vi "Airmar open and config serial port.vi"(8 "error in (no error)":errorcluster, 9 "Input\nbuffer size":u32=4096, 10 "baud rate":u32=4800, 11 "VISA Refnum in":refnum<visa-resource-name>) -> (0 "error out":errorcluster, 3 "VISA Refnum out":refnum<visa-resource-name>)   [LabVIEW 2013]
doc: "opens a serial port (on the RIO or a standard computer) and sets up the buffers so they actually work.\n-Jason"
uses:
  <vilib>/Instr/_visa.llb/VISA Configure Serial Port (Instr).vi
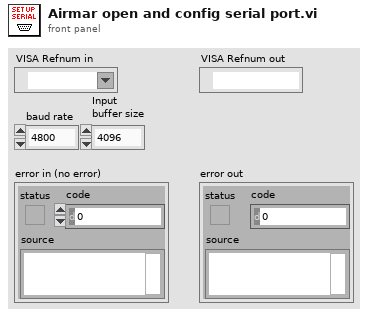
[diagram p1: front panel]
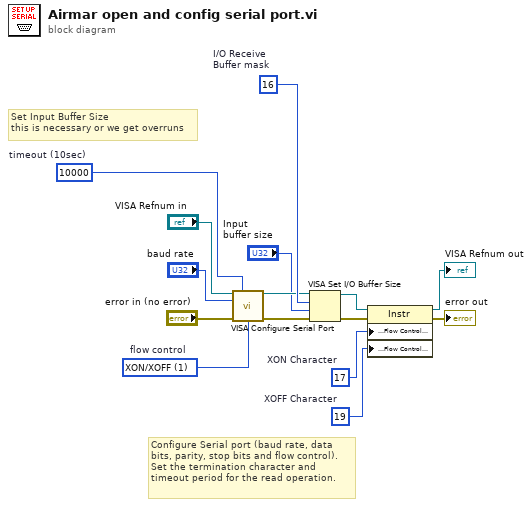
[diagram p0: block diagram]
diagram:
  w10 = u32 10000  # timeout (10sec)
  w7 = u8 19  # XOFF Character
  w6 = u8 17  # XON Character
  w11 = u16 16  # I/O Receive Buffer mask
  w2 = u16 1 items=["None"=0, "XON/XOFF"=1, "RTS/CTS"=2, "DTR/DSR"=4]  # flow control
  # "Set Input Buffer Size\nthis is necessary or we get overruns"
  # "Configure Serial port (baud rate, data\nbits, parity, stop bits and flow control).\nSet the termination character and\ntimeout period for the read operation."
  n1 = call-poly "VISA Configure Serial Port"("VISA resource name"="VISA Refnum in", "timeout (10sec)"=w10, "baud rate (9600)"="baud rate", "error in (no error)"="error in (no error)", "flow control (0:none)"=w2) -> ("VISA resource name out"=w8:refnum<visa-resource-name>, "error out"=w9:errorcluster)  [unwired: 9 in]
  n2 = VISA Set I/O Buffer Size(VISA resource name=w8, mask (16)=w11, size (4096)="Input\nbuffer size", error in (no error)=w9) -> (VISA resource name out=w4:refnum<visa-resource-name>, error out=w5:errorcluster)
  n3 = property class="Instr"(reference=w4, error in=w5, "Serial Settings:Flow Control XON Character"=w6, "Serial Settings:Flow Control XOFF Character"=w7) -> (reference out=→"VISA Refnum out":refnum<visa-resource-name>, error out=→"error out":errorcluster)
